vi "Report Raw Data.vi"(9 "Data":T1={"Datetime"="DateTime", "User Name"="Barcode", "Running Model"="Operator_Name", "Barcode"="Operator_Name", "Barcode difusser"="Operator_Name"}, 10 "Sensor Data":T2={"Load Min(N)"="Load min(N)", "Load Max(N)"="Load max(N)", "Load(N) "="Load (N)", "Dist Min(mm)"="Dist min(mm)", "Dist Max(mm)"="Dist max(mm)", "Dist (mm)"="Dist (mm)", "Load Status"="Load Status", "Dist Status"="Dist Status"}, 11 "test":string[][](array[string])=[["1", "Light Box Ionization", "Pass"], ["2", "Light box Clamp", "Pass"], ["3", "Difusser Put on Light Box", "Pass"], ["4", "Photo Prism Put On LB", "Test In Progress"], ["5", "LCD Put On Light Box", ""], ["6", "Difusser Checking Position", ""], ["7", "Adesive Tap check Camera", ""], ["8", "LCD Placing Position", ""], ["9", "Camera check Adhesive Taps", ""], ["10", "LCD Display Rotating ", ""], ["11", "Camera Slide Unit", ""], ["12", "LCD Pressing Servo", ""], ["13", "LCD Pressing servo up", ""], ["14", "Camera Unit Rev", ""], ["15", "Fixture Slide Up", ""], ["16", "Light Box Unclamp", ""]]) -> (2 "Data":string[](array[string]), 3 "Header":string[](array[string]))   [LabVIEW 2015]
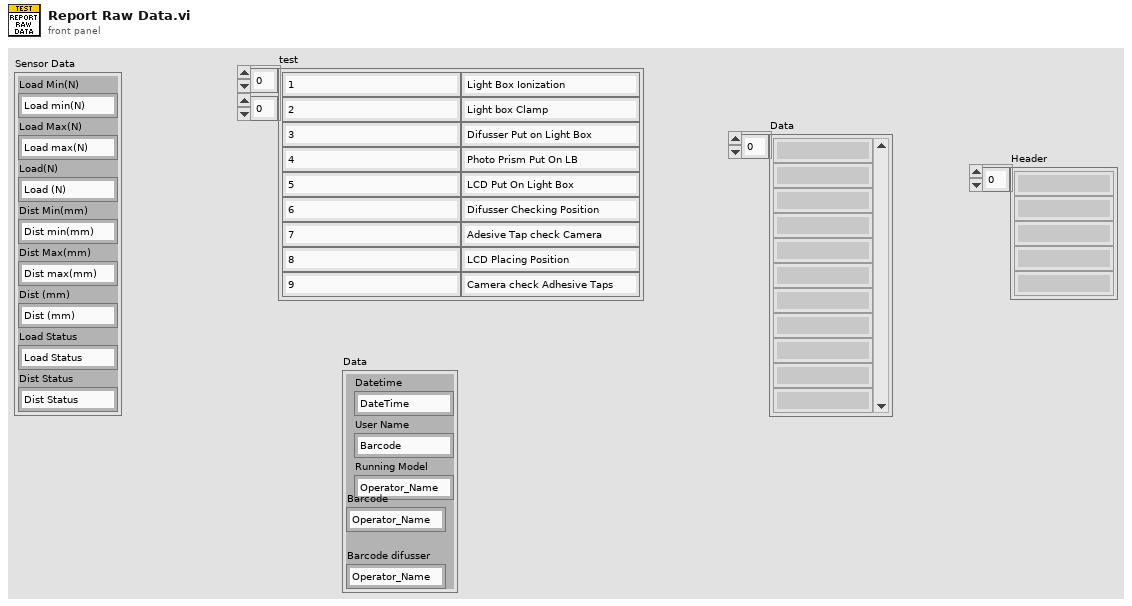
[diagram p1: front panel]
types:
  T1 = cluster{"Datetime":string, "User Name":string, "Running Model":string, "Barcode":string, "Barcode difusser":string}
  T2 = cluster{"Load Min(N)":string, "Load Max(N)":string, "Load(N) ":string, "Dist Min(mm)":string, "Dist Max(mm)":string, "Dist (mm)":string, "Load Status":string, "Dist Status":string}
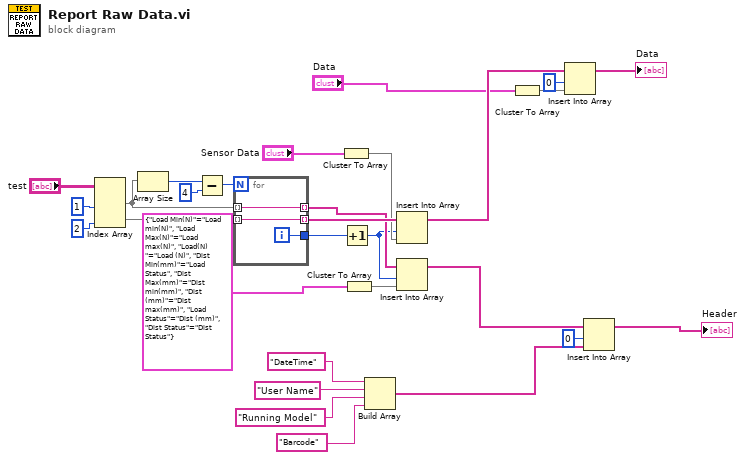
[diagram p0: block diagram]
diagram:
  n1 = Index Array(array="test", index (col) #1=1 ("disabled index (col)"), index (col) #2=2 ("index (col)")) -> (element #1=w26:string[], element #2=w22:string[])  [unwired: 2 in]
  n2 = Array Size(array=w26) -> (size(s)=w25:i32)
  n3 = Subtract(x=w25, y=4) -> (x-y=w23:i32)
  n4 = for {
    N: w23 -> [_]
    tunnel: w26 -> [w32] mode=indexing
    tunnel: w22 -> [w31] mode=indexing
    tunnel: [w32] -> w17 mode=indexing
    tunnel: [w31] -> w21 mode=indexing
    tunnel: [w30] -> w20
    i -> [w30]
  }
  n5 = Cluster To Array(cluster="Sensor Data") -> (array=w19:string[])
  n6 = Increment(x=w20) -> (x+1=w16:i32)
  n7 = Cluster To Array(cluster=T2 {"Load Min(N)"="Load min(N)", "Load Max(N)"="Load max(N)", "Load(N) "="Load (N)", "Dist Min(mm)"="Load Status", "Dist Max(mm)"="Dist min(mm)", "Dist (mm)"="Dist max(mm)", "Load Status"="Dist (mm)", "Dist Status"="Dist Status"} ("Sensor Data 2")) -> (array=w15:string[])
  n8 = Build Array("DateTime", "User Name" ("element"), "Running Model" ("element"), "Barcode" ("element")) -> (w8:string[])
  n9 = Insert Into Array(array=w21, index=w16, new element=w19) -> (w6:string[])
  n10 = Insert Into Array(array=w17, index=w16, new element=w15) -> (w9:string[])
  n11 = Cluster To Array(cluster="Data") -> (array=w3:string[])
  n12 = Insert Into Array(array=w6, index=0, new element=w3) -> (→"Data":string[])
  n13 = Insert Into Array(array=w9, index=0, new element=w8) -> (→"Header":string[])
